vi "HeaderAction.vi"(0 "DefaultDevIn":refnum<class "AppliedMotionDrive.lvclass"> caption="DNL_LabVIEW Object in", 11 "error in (no error)":errorcluster caption="entrée d'erreur (pas d'erreur)") -> (4 "DefaultDevOut":refnum<class "AppliedMotionDrive.lvclass"> caption="DNL_LabVIEW Object out", 6 "DataNames":string[](array[string]), 8 "Instr Name":string, 10 "HeaderString":string, 13 "ArrDatNames":string[](array[string]), 14 "DisplayNames":string[](array[string]), 15 "error out":errorcluster caption="sortie d'erreur")   [LabVIEW 2019, in "AppliedMotionDrive.lvclass"]
uses:
  AppliedMotionDrive.lvclass
  C:/Programmes Labview/LabscanV1A/DevicesClass/BaseDevice/BaseDevice.lvclass
  AppliedMotionDrive.lvclass/AppliedMotionDrive.ctl
  BaseDevice/BaseDevice.lvclass
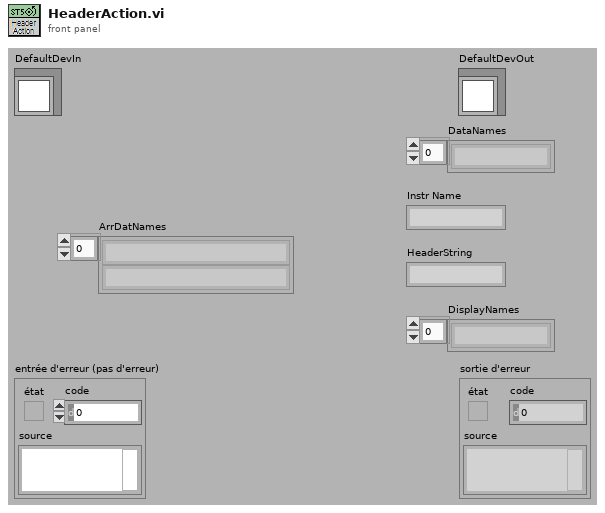
[diagram p1: front panel]
types:
  T1 = typedef "AppliedMotionDrive.lvclass/AppliedMotionDrive_Func.ctl" = enum16{"Position (Units)", "FilterWheel (Id)"}
  T2 = cluster{"Enabled":bool, "Sampling":bool, "Fault":bool, "In Position":bool, "Moving":bool, "Jogging":bool, "Stopping":bool, "Wait Input":bool, "Saving":bool, "Alarm":bool, "Homing":bool, "Waiting":bool, "Wait Time":bool, "Wizard":bool, "Checking Enc":bool, "Q mode":bool, "Initializing":bool}
  T3 = cluster{"Vitesse (Tour/s)":dbl, "Accél":dbl, "Décél":dbl, "Accél Max":dbl, "Idle Current (A) ":dbl}
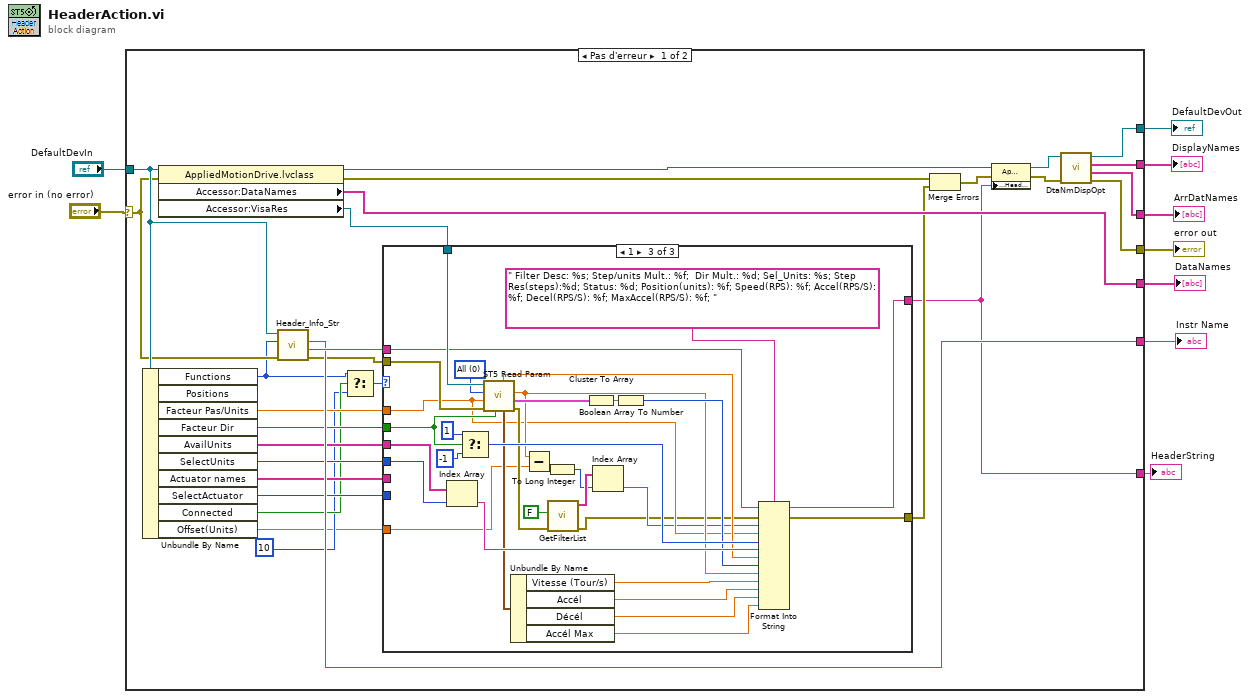
[diagram p0: block diagram]
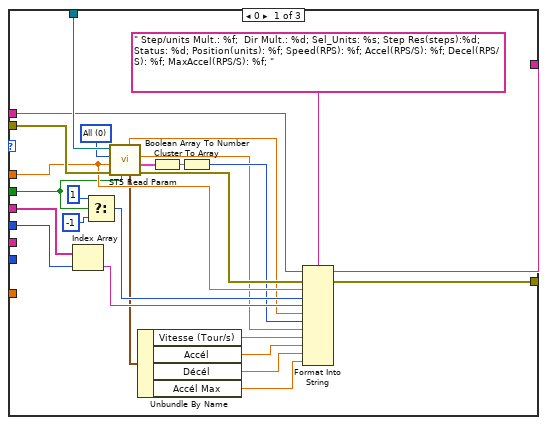
[diagram p2: hidden frame]
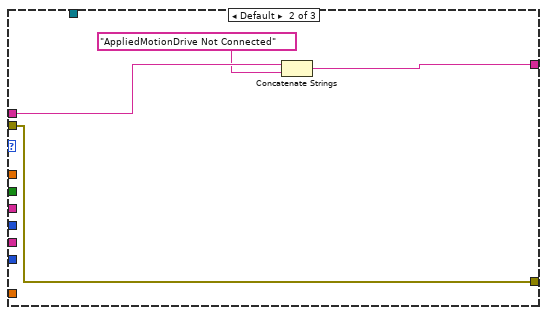
[diagram p3: hidden frame]
diagram:
  n1 = case shown="Pas d'erreur" "error in (no error)" {
    selector: "error in (no error)" -> [w32 w102]
    tunnel: [w15 _] -> w8
    tunnel: [w18 _] -> w7
    tunnel: "DefaultDevIn" -> [w33 w103]
    tunnel: [w17 w102] -> w5
    tunnel: [w30 w103] -> w4
    tunnel: [w27 _] -> w3
    tunnel: [w34 _] -> w2
    tunnel: [w29 _] -> w1
    frame No Error {
      n2 = Unbundle By Name(w33) -> ("Functions"=w12:T1, "Facteur Pas/Units"=w26:dbl, "Facteur Dir"=w25:bool, "AvailUnits"=w24:string[], "SelectUnits"=w23:u8, "Actuator names"=w22:string[], "SelectActuator"=w21:u8, "Connected"=w13:bool, "Offset(Units)"=w10:dbl)  [unwired: 1 out]
      n3 = property class="AppliedMotionDrive.lvclass"(reference=w33, error in=w32) -> (reference out=w38:refnum<class "AppliedMotionDrive.lvclass">, error out=w37:errorcluster, "Accessor:DataNames"=w18:string[], "Accessor:VisaRes"=w20:refnum<visa-resource-name>)
      n4 = call-dynamic "Header_Info_Str.vi"("error in (no error)"=w32, "Functions"=w12, "DefaultDev in"=w33) -> ("error out"=w19:errorcluster, "HdrInfoStr"=w28:string, "InstrumentName"=w27:string)  [unwired: 5 in, 1 out]
      n5 = Select(t=w12, s=w13, f=u16 10) -> (s? t:f=w14:u16)
      n6 = case shown="1" w14 {
        tunnel: [w52 w66 w90] -> w15
        tunnel: w28 -> [w53 w67 w91]
        tunnel: w26 -> [w55 _ w73]
        tunnel: w25 -> [w45 _ w85]
        tunnel: w24 -> [w58 _ w95]
        tunnel: w23 -> [w57 _ w94]
        tunnel: w22 -> [_ _ _]
        tunnel: w21 -> [_ _ _]
        tunnel: w20 -> [w64 _ w101]
        tunnel: w19 -> [w63 w68 w100]
        tunnel: [w39 w68 w79] -> w16
        tunnel: w10 -> [_ _ w69]
        frame 0 {
          w62 = u16 0 items=["All", "Velocity", "Acceleration", "Deceleration", "Max Acceleration", "Position", "Step/Rev", "Alarm Code", "Status"] ("Parameters")
          n7 = Index Array(array=w58, index=w57) -> (element=w54:string)
          n8 = Select(t=1 ("pas/mm"), s=w45, f=-1 ("pas/mm")) -> (s? t:f=w56:i32)
          n9 = call <userlib>:"ST5 Read Param.vi"("Facteur Dir"=w45, "error in (no error)"=w63, "Facteur Pas"=w55, "Parameters"=w62, "Port COM"=w64) -> ("error out"=w51:errorcluster, "Status"=w50:T2, "Position"=w47:dbl, "Speed Par"=w46:T3, "Résolution Pas"=w44:dbl)  [unwired: 2 out]
          n10 = Unbundle By Name(w46) -> ("Vitesse (Tour/s)"=w43:dbl, "Accél"=w42:dbl, "Décél"=w41:dbl, "Accél Max"=w40:dbl)
          n11 = Cluster To Array(cluster=w50) -> (array=w49:bool[])
          n12 = Boolean Array To Number(Boolean array=w49) -> (number=w48:u32)
          n13 = Format Into String(format string=" Step/units Mult.: %f;  Dir Mult.: %d; Sel_Units: %s; Step Res(steps):%d; Status: %d; Position(units): %f; Speed(RPS): %f; Accel(RPS/S): %f; Decel(RPS/S): %f; MaxAccel(RPS/S): %f; " ("chaîne de format"), initial string=w53, error in=w51, w55, w56, w54, w44, w48, w47, w43, w42, w41, w40) -> (resulting string=w52:string, error out=w39:errorcluster)
        }
        frame Default {
          n14 = Concatenate Strings(w67, "AppliedMotionDrive Not Connected" ("chaîne")) -> (w66:string)
        }
        frame 1 {
          w99 = u16 0 items=["All", "Velocity", "Acceleration", "Deceleration", "Max Acceleration", "Position", "Step/Rev", "Alarm Code", "Status"] ("Parameters")
          n15 = Index Array(array=w95, index=w94) -> (element=w92:string)
          n16 = Select(t=1 ("pas/mm"), s=w85, f=-1 ("pas/mm")) -> (s? t:f=w93:i32)
          n17 = call <userlib>:"ST5 Read Param.vi"("Facteur Dir"=w85, "error in (no error)"=w100, "Facteur Pas"=w73, "Parameters"=w99, "Port COM"=w101) -> ("error out"=w77:errorcluster, "Status"=w89:T2, "Position"=w76:dbl, "Speed Par"=w86:T3, "Résolution Pas"=w84:dbl)  [unwired: 2 out]
          n18 = Unbundle By Name(w86) -> ("Vitesse (Tour/s)"=w83:dbl, "Accél"=w82:dbl, "Décél"=w81:dbl, "Accél Max"=w80:dbl)
          n19 = Subtract(x=w76, y=w69) -> (x-y=w70:dbl)
          n20 = To Long Integer(number=w70) -> (32bit integer=w74:i32)
          n21 = call "GetFilterList.vi"("Error in"=w77, "Write"=FALSE) -> ("Error out"=w71:errorcluster, "Filter names out"=w75:string[])  [unwired: 4 in]
          n22 = Cluster To Array(cluster=w89) -> (array=w88:bool[])
          n23 = Index Array(array=w75, index=w74) -> (element=w72:string)
          n24 = Boolean Array To Number(Boolean array=w88) -> (number=w87:u32)
          n25 = Format Into String(format string=" Filter Desc: %s; Step/units Mult.: %f;  Dir Mult.: %d; Sel_Units: %s; Step Res(steps):%d; Status: %d; Position(units): %f; Speed(RPS): %f; Accel(RPS/S): %f; Decel(RPS/S): %f; MaxAccel(RPS/S): %f; " ("chaîne de format"), initial string=w91, error in=w71, w72, w73, w93, w92, w84, w87, w76, w83, w82, w81, w80) -> (resulting string=w90:string, error out=w79:errorcluster)
        }
      }
      n26 = Merge Errors(w37, w16) -> (w31:errorcluster)
      n27 = property class="AppliedMotionDrive.lvclass"(reference=w38, error in=w31, "Accessor:HeaderString"=w15) -> (reference out=w35:refnum<class "AppliedMotionDrive.lvclass">, error out=w36:errorcluster)
      n28 = call "DtaNmDispOpt.vi"("error in (no error)"=w36, "BaseDevice en entrée"=w35) -> ("error out"=w17:errorcluster, "ArrDisplayNames"=w29:string[], "DisplayNames"=w34:string[], "BaseDevice en sortie"=w30:refnum<class "AppliedMotionDrive.lvclass">)  [unwired: 6 in]
    }
    frame Error {
    }
  }
  "error out" <- w5
  "DefaultDevOut" <- w4
  "DataNames" <- w7
  "HeaderString" <- w8
  "Instr Name" <- w3
  "DisplayNames" <- w2
  "ArrDatNames" <- w1
